vi "VS_OpenStimProfileMngRef.vi"(0 "Engine Reference(in)":refnum<k7>, 1 "Condition Run?":bool, 5 "Sequence File Ref(in)":refnum<k7>, 7 "VeriStand version info":T1={"VeriStand.exe Path"="", "Assembly"="", "Constructor Token"=0, "Module Token"={"GetIWorkspaceToken"=100663761, "GetIStimulusToken"=100663772, "GetIModelManagerToken"=100663768, "GetIProjectToken"=100663780, "RunProjectToken"=100663643, "CloseProjectToken"=100663640, "RunWorkspaceToken"=100663694, "StopWorkspaceToken"=100663695, "SetSingleChannelToken"=100663609, "SetMultipleParametersToken"=100663608, "RunStimulusToken"=100663670, "GetStimulusStateToken"=100663669, "Open WorkspaceToken"=0, "DeployToken"=0, "UndeployToken"=0, "QuitToken"=0}}, 11 "error in":errorcluster, 12 "Step Group":i32(ring) items=["StepGroup_Setup", "StepGroup_Main", "StepGroup_Cleanup"], 13 "Step Index":i32) -> (4 "Engine reference(out)":refnum<k7>, 6 "Sequence File Ref(out)":refnum<k7>, 8 "VeriStand version info (out)":T1={"VeriStand.exe Path"="", "Assembly"="", "Constructor Token"=0, "Module Token"={"GetIWorkspaceToken"=100663761, "GetIStimulusToken"=100663772, "GetIModelManagerToken"=100663768, "GetIProjectToken"=100663780, "RunProjectToken"=100663643, "CloseProjectToken"=100663640, "RunWorkspaceToken"=100663694, "StopWorkspaceToken"=100663695, "SetSingleChannelToken"=100663609, "SetMultipleParametersToken"=100663608, "RunStimulusToken"=100663670, "GetStimulusStateToken"=100663669, "Open WorkspaceToken"=0, "DeployToken"=0, "UndeployToken"=0, "QuitToken"=0}}, 15 "error out":errorcluster)   [LabVIEW 2010]
doc: "This VI creates the VeriStand object reference step in TestStand to access the dotNet API. This VI needs to be called always at the beginning of any VeriStand sequence in TestStand"
uses:
  Ctls/dotNetAssemblyInfo.ctl
  Ctls/VSModuleTokens.ctl
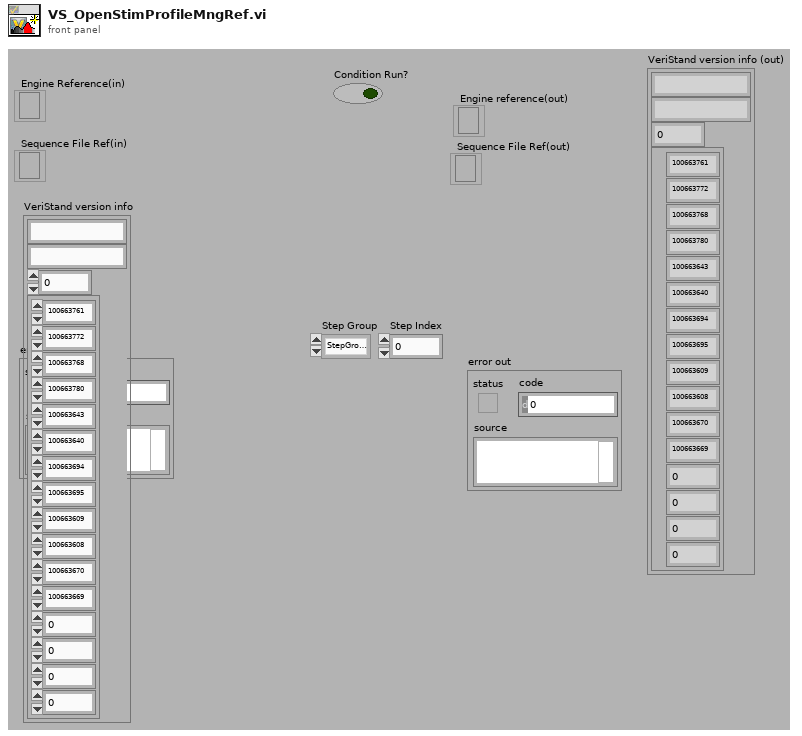
[diagram p1: front panel]
types:
  T1 = typedef "dotNetAssemblyInfo.ctl" = cluster{"VeriStand.exe Path":string, "Assembly":string, "Constructor Token":i32, "Module Token":T2}
  T2 = typedef "VSModuleTokens.ctl" = cluster{"GetIWorkspaceToken":i32, "GetIStimulusToken":i32, "GetIModelManagerToken":i32, "GetIProjectToken":i32, "RunProjectToken":i32, "CloseProjectToken":i32, "RunWorkspaceToken":i32, "StopWorkspaceToken":i32, "SetSingleChannelToken":i32, "SetMultipleParametersToken":i32, "RunStimulusToken":i32, "GetStimulusStateToken":i32, "Open WorkspaceToken":i32, "DeployToken":i32, "UndeployToken":i32, "QuitToken":i32}
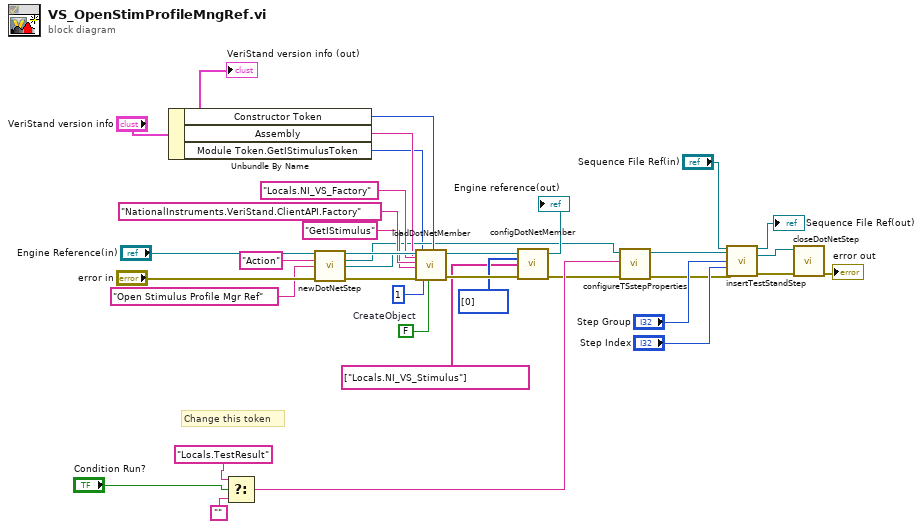
[diagram p0: block diagram]
diagram:
  w19 = FALSE  # CreateObject
  # "Change this token"
  n1 = Unbundle By Name("VeriStand version info") -> ("Constructor Token"=w13:i32, "Assembly"=w14:string, "Module Token.GetIStimulusToken"=w1:i32)
  n2 = Select(t="Locals.TestResult", s="Condition Run?", f="") -> (s? t:f=w5:string)
  n3 = call "newDotNetStep.vi"("Engine reference"="Engine Reference(in)", "stepType"="Action", "Step Name"="Open Stimulus Profile Mgr Ref", "error in"="error in") -> ("Engine reference(out)"=→"Engine reference(out)":refnum<k7>, "NewStep (out)"=w7:refnum<k7>, "dotNetModule(out)"=w23:refnum<k7>, "error out"=w35:errorcluster)  [unwired: 8 in]
  n4 = call "loadDotNetMember.vi"("dotNetModule"=w23, "Strong Assembly path"=w14, "ClassName"="NationalInstruments.VeriStand.ClientAPI.Factory", "MemberName"="GetIStimulus", "Member token"=w1, "error in(no error)"=w35, "ClassReference"="Locals.NI_VS_Factory", "Call Member?"=1 ("Call Memeber?"), "CreateObject"=w19, "Constructor Token"=w13) -> ("dotNetModule(out)"=w18:refnum<k7>, "error out"=w17:errorcluster)  [unwired: 8 in]
  n5 = call "configDotNetMember.vi"("dotNetModule"=w18, "Index array"=i32[] [0], "Parameter Value array"=string[] ["Locals.NI_VS_Stimulus"], "error in (no error)"=w17) -> ("error out"=w4:errorcluster)  [unwired: 11 in]
  n6 = call "configureTSstepProperties.vi"("error in"=w4, "Precondition"=w5, "NewStep (in)"=w7) -> ("error out"=w3:errorcluster, "NewStep (out)"=w6:refnum<k7>)  [unwired: 7 in]
  n7 = call "insertTestStandStep.vi"("Sequence File Ref"="Sequence File Ref(in)", "Step to insert"=w6, "Step Group"="Step Group", "index"="Step Index", "error out"=w3) -> ("Sequence File Ref(out)"=→"Sequence File Ref(out)":refnum<k7>, "Step to insert (out)"=w34:refnum<k7>, "error out"=w32:errorcluster)  [unwired: 8 in]
  n8 = call "closeDotNetStep.vi"("error in"=w32, "NewStep"=w34) -> ("error out"=→"error out":errorcluster)  [unwired: 9 in]
  "VeriStand version info (out)" <- "VeriStand version info"
